vi "Read SamplesPerCycle.vi"(8 "error in (no error)":errorcluster, 11 "nCRD in":refnum<class "gCRD.lvclass">) -> (0 "error out":errorcluster, 2 "SamplesPerCycle":u16, 3 "nCRD out":refnum<class "gCRD.lvclass">)   [LabVIEW 2016, in "gCRDS.lvlib" / "gCRD.lvclass"]
uses:
  gCRD.lvclass
  gCRD.lvclass/gCRD.ctl
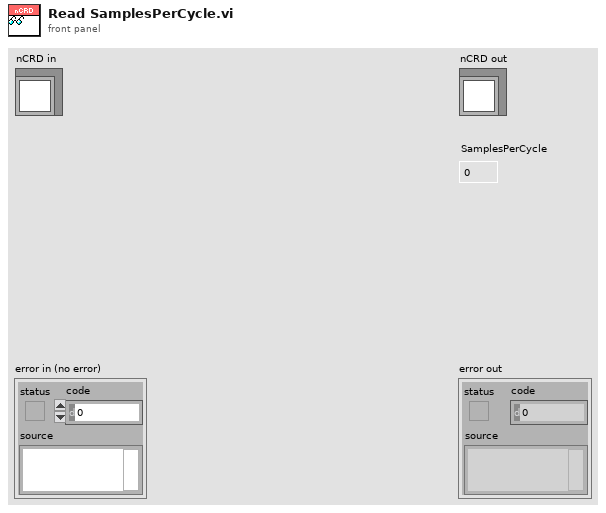
[diagram p1: front panel]
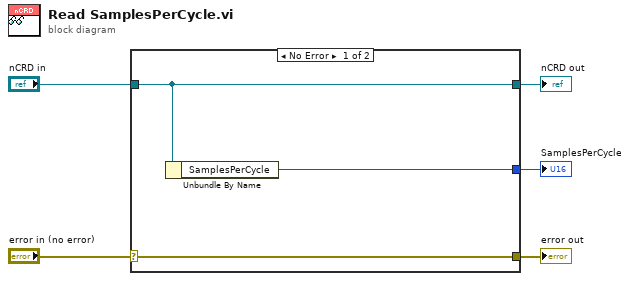
[diagram p0: block diagram]
diagram:
  n1 = case shown="No Error" "error in (no error)" {
    selector: "error in (no error)" -> [w8 w9]
    tunnel: [w8 w9] -> w4
    tunnel: [w7 w10] -> w2
    tunnel: "nCRD in" -> [w7 w10]
    tunnel: [w6 _] -> w1
    frame No Error {
      n2 = Unbundle By Name(w7) -> ("SamplesPerCycle"=w6:u16)
    }
    frame Error {
    }
  }
  "error out" <- w4
  "nCRD out" <- w2
  "SamplesPerCycle" <- w1
